vi "Random Seas.vi"() -> ()   [LabVIEW 2012]
uses:
  <vilib>/Daq/1easyio.llb/AO Update Channel (scaled value).vi
  Instance           1 19Saved   Random Seas .vi
  Instance           2 19Saved   Random Seas .vi
panel:
  out "File Name Out":path
  out "Wavestaff Signal":dbl[](graph)
  in  "Measure Waves":bool
  in  "Input Settings":bool
  in  "Geometric Settings":bool
  in  "Limit Settings":bool
  in  "Output Settings":bool
  out "Output Sig. Wave Height":dbl format="%.4f"
  out "Buffer Completed":dbl format="%.1f"
  out "Time Series Data":dbl[](array[numeric]) format="%.2f"
  out "Output Signal":dbl[](graph)
  in  "Set spectal parameters":bool
  in  "Run":bool
  in  "Power":bool
  out "Significant Wave Period":dbl format="%.4f"
  out "Significant Wave Height":dbl format="%.4f"
  in  "Select spectrum":u16(ring) items=["Bretschnieder", "JONSWAP", "NH Extreme", "NH Typical", "Pierson Moskowitz"]
  out "Spectra":cluster{"Numeric":dbl, "Numeric":dbl}[](graph)
  out "Time Series":cluster{"Numeric":dbl, "Numeric":sgl}[](graph)
  # "Random Sea Generator"
  # "m"
  # "s"
  # "Time (min:sec)"
  # "%"
  # "m"
  # "Time (min:sec)"
  # "Frequency (Hz)"
  # "Advanced"
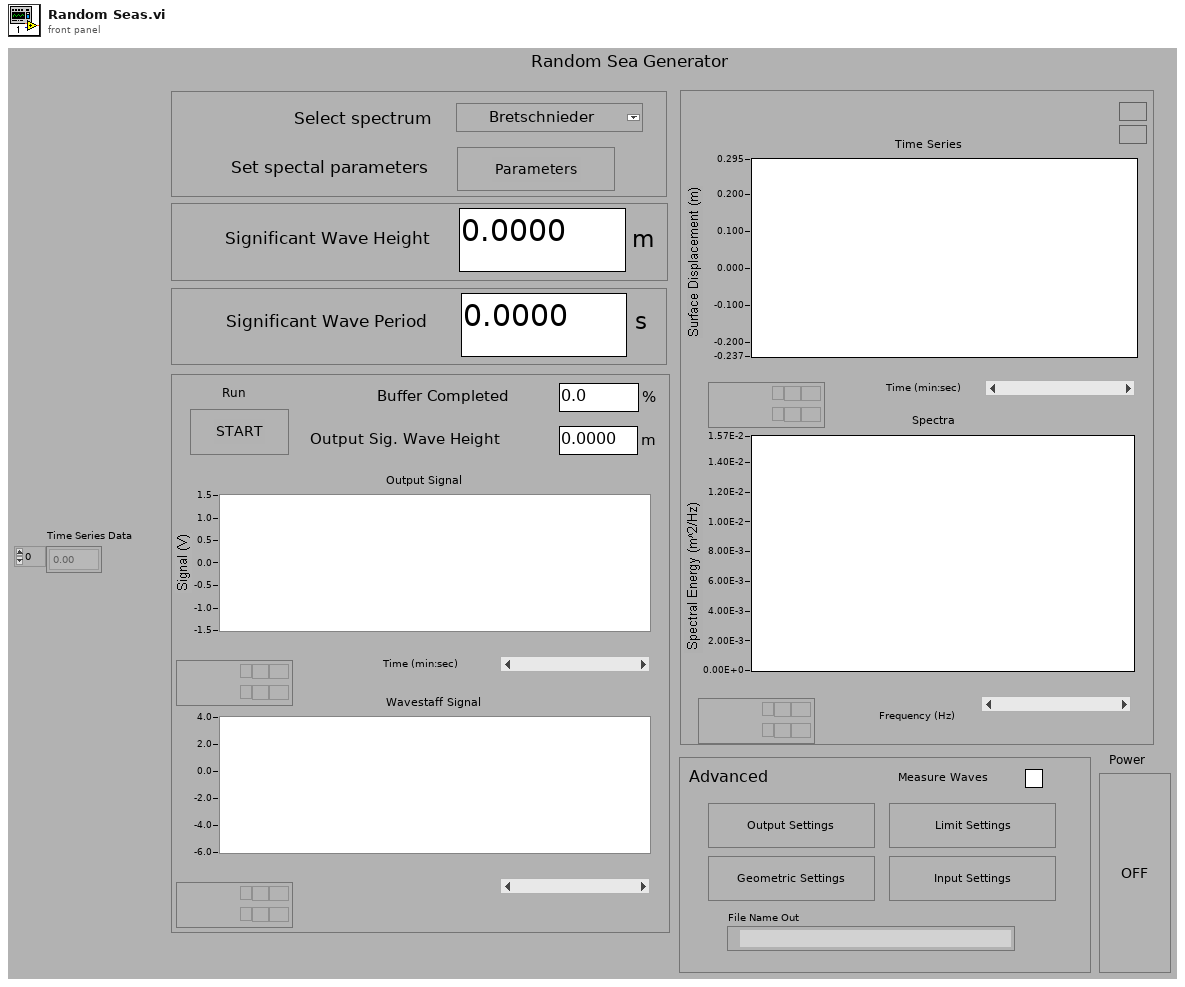
[diagram p1: front panel]
types:
  T1 = cluster{"Input Device":i32, "Input Channel":string, "Input Offset":dbl, "Input Calibration":dbl}
  T2 = cluster{"Device":i16, "Channel":string, "Sampling Rate":i32, "Ramp Time":dbl, "Buffer Length":u16, "Buffer Size":i32, "Sub Buffer Length":i16, "Sub Buffer Size":i16}
  T3 = cluster{"Stroke Calibration":dbl, "Water Depth":dbl, "Paddle Height":dbl}
  T4 = cluster{"Min Wave Period":dbl, "Max Wave Period":dbl, "Cutoff Frequency":dbl, "Max 1/2 Piston Stroke":dbl, "Max H/L":dbl, "Max H/d":dbl}
  T5 = cluster{"Bretschneider":cluster{"Sig Wave Height":dbl, "Sig Wave Period":dbl, "Scale Ratio":dbl}, "JONSWAP":cluster{"Sig Wave Height":dbl, "Sig Wave Period":dbl, "Gamma":dbl, "Sigma A":dbl, "Sigma B":dbl, "Scale Ratio":dbl}, "NH Extreme":cluster{"Sig Wave Height":dbl, "Sig Wave Period":dbl, "Gamma":dbl, "Sigma A":dbl, "Sigma B":dbl, "P":dbl, "Scale Ratio":dbl}, "NH Typical":cluster{"Sig Wave Height":dbl, "Sig Wave Period 1":dbl, "Sig Wave Period 2":dbl, "Gamma 1":dbl, "Gamma 2":dbl, "P":dbl, "Scale Ratio":dbl}, "PM":cluster{"Wind speed":dbl, "Scale Ratio":dbl}}
  T6 = cluster{"Element Data":dbl, "Element Data":dbl}[]
  T7 = cluster{"Sig Wave Height":dbl, "Sig Wave Period":dbl, "Scale Ratio":dbl}
  T8 = cluster{"Sig Wave Height":dbl, "Sig Wave Period":dbl, "Gamma":dbl, "Sigma A":dbl, "Sigma B":dbl, "Scale Ratio":dbl}
  T9 = cluster{"Sig Wave Height":dbl, "Sig Wave Period":dbl, "Gamma":dbl, "Sigma A":dbl, "Sigma B":dbl, "P":dbl, "Scale Ratio":dbl}
  T10 = cluster{"Sig Wave Height":dbl, "Sig Wave Period":dbl, "Sig Wave Period 2":dbl, "Gamma 1":dbl, "Gamma 2":dbl, "P":dbl, "Scale Ratio":dbl}
  T11 = cluster{"Device":i16, "Channel":string, "Sampling Rate":i32, "Stroke Calibration":dbl, "Buffer Length":u16, "Buffer Size":i32, "Sub Buffer Length":i16, "Sub Buffer Size":i16}
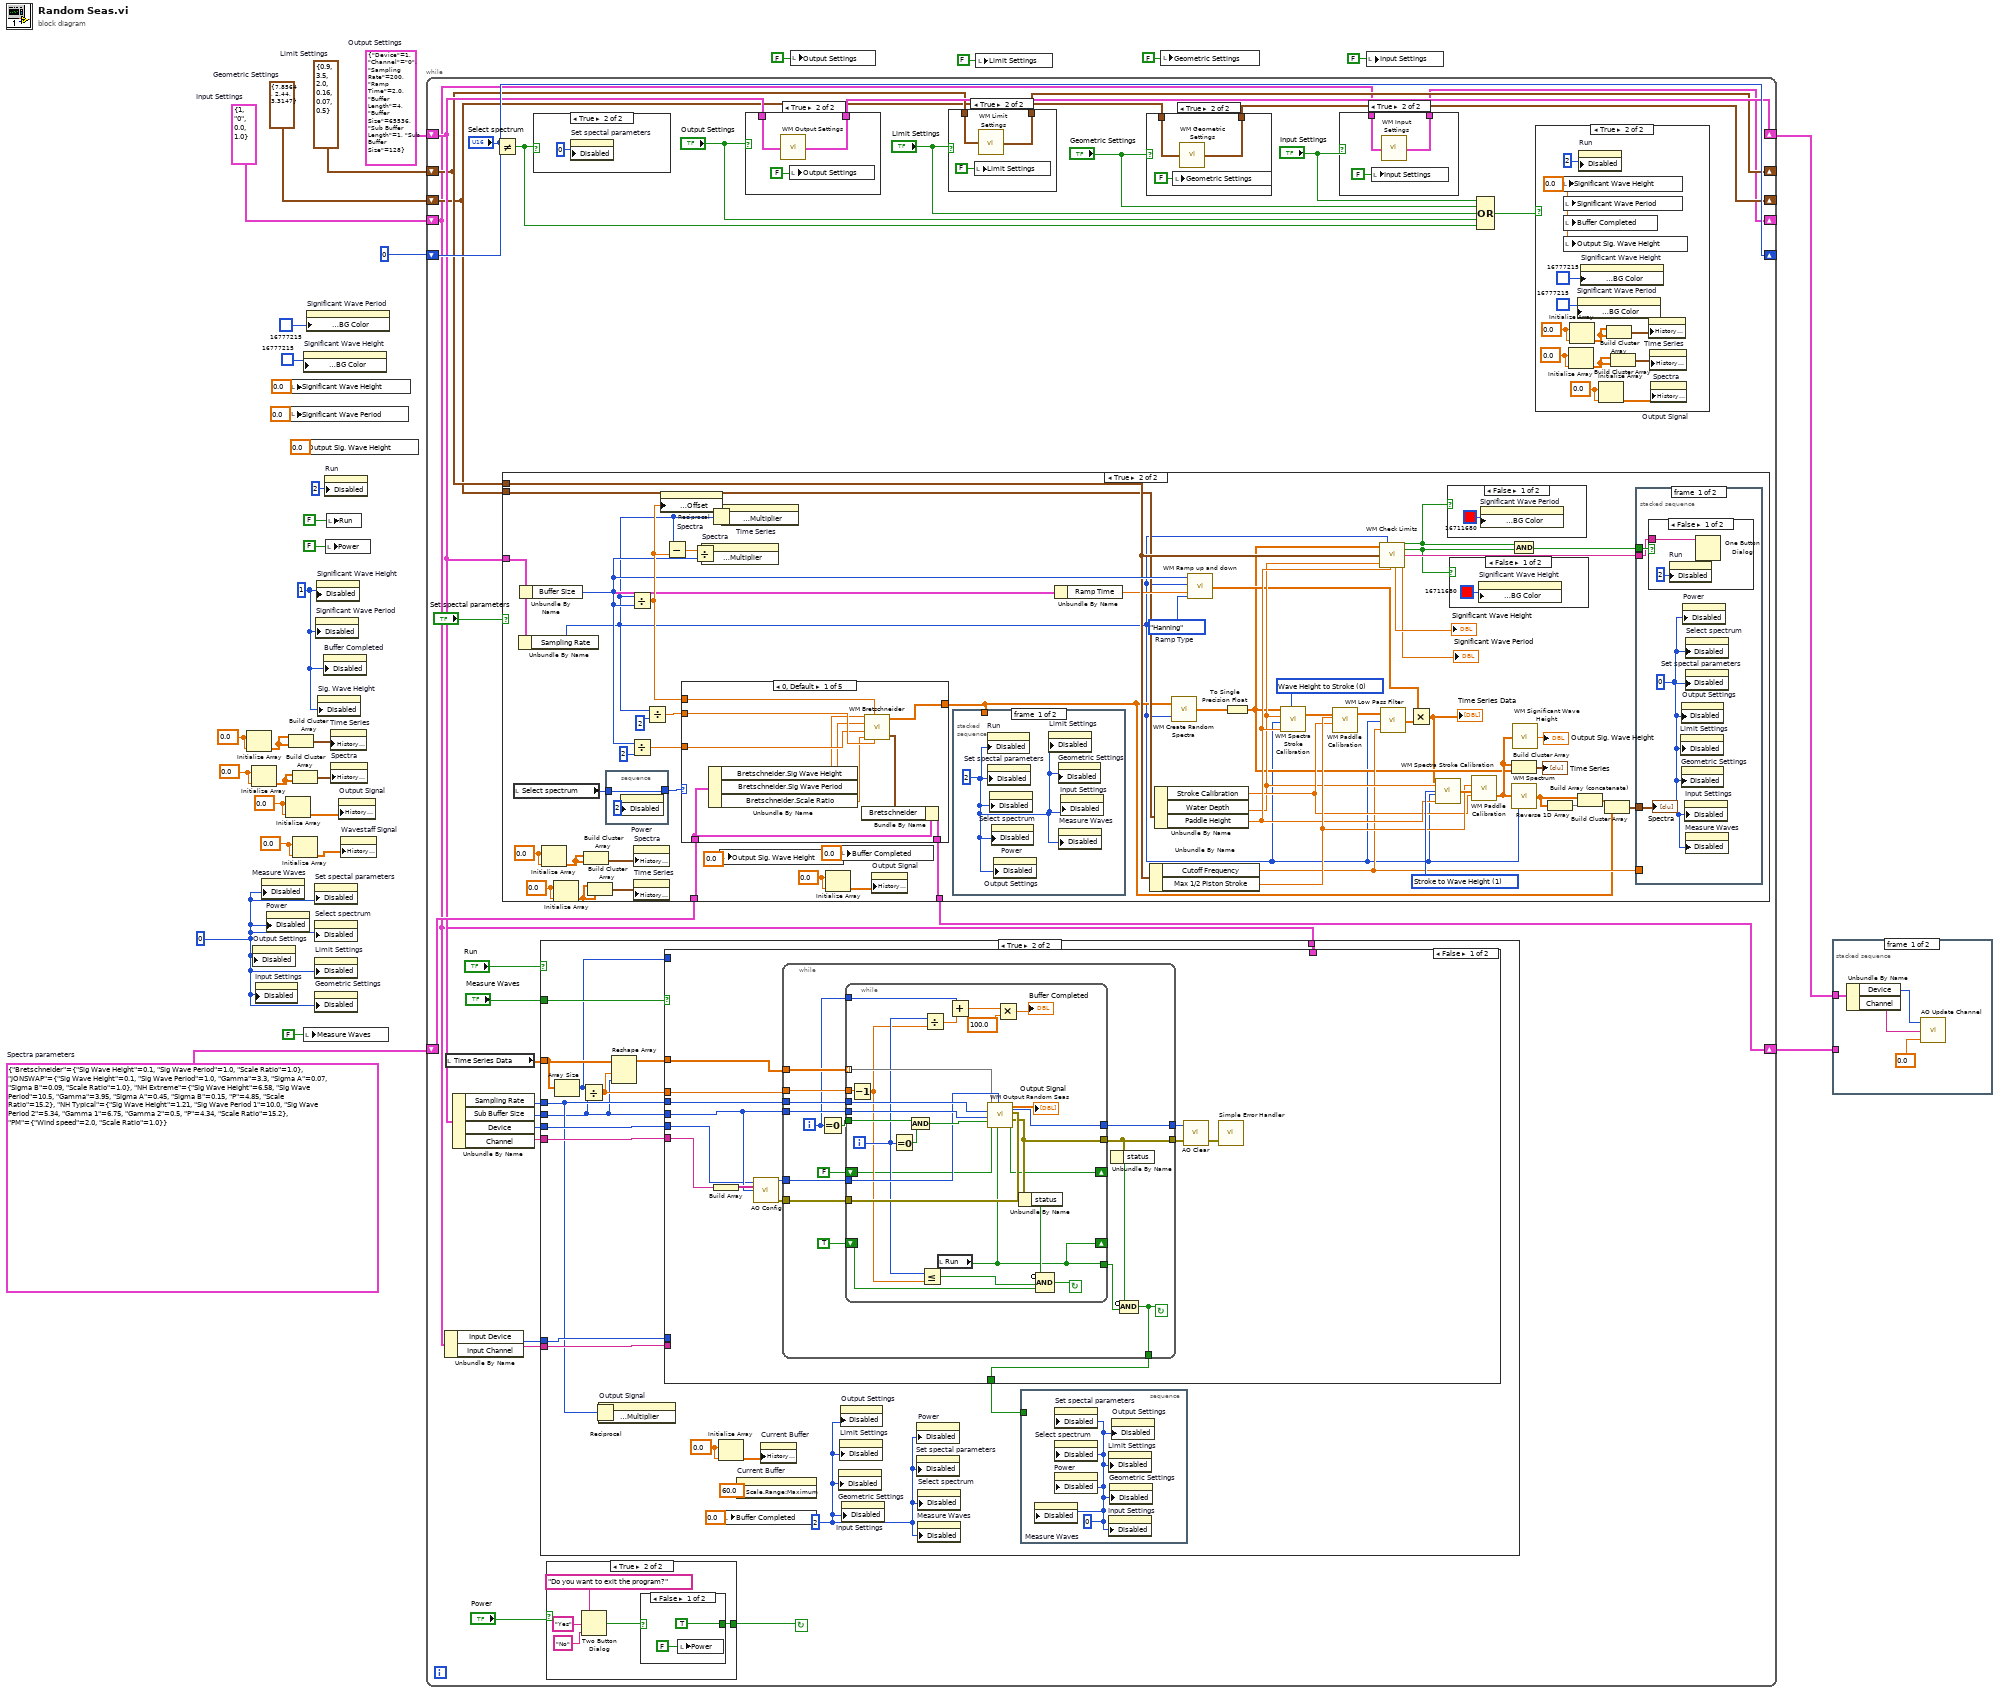
[diagram p0: block diagram]
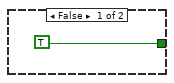
[diagram p7: hidden frame]
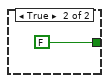
[diagram p8: hidden frame]
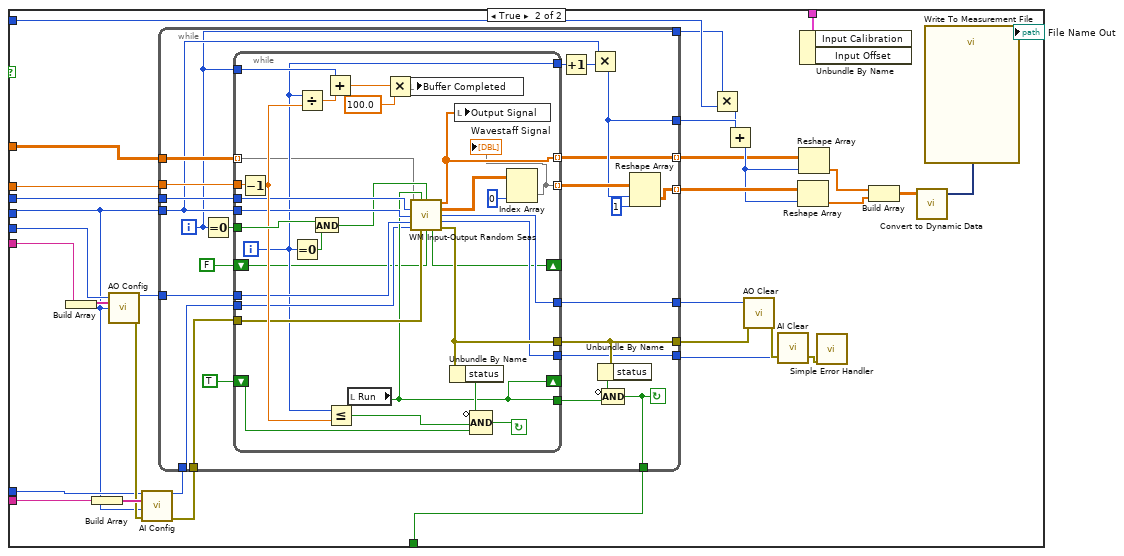
[diagram p11: hidden frame]
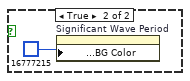
[diagram p13: hidden frame]
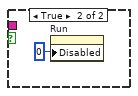
[diagram p15: hidden frame]
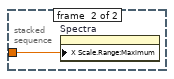
[diagram p16: hidden frame]
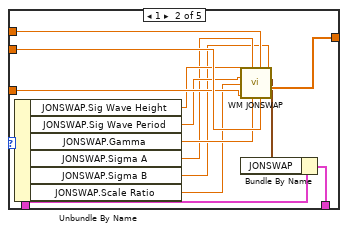
[diagram p17: hidden frame]
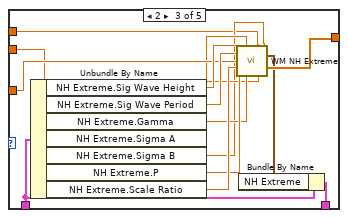
[diagram p18: hidden frame]
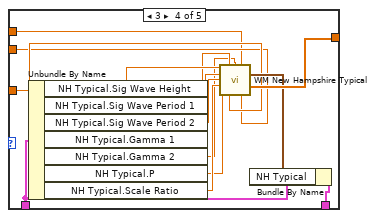
[diagram p19: hidden frame]
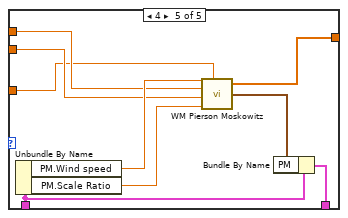
[diagram p20: hidden frame]
diagram:
  w2 = 0.0 ("Element Data")
  w5 = T1 {"Input Device"=1, "Input Channel"="0", "Input Offset"=0.0, "Input Calibration"=1.0}  # Input Settings
  w8 = T2 {"Device"=1, "Channel"="0", "Sampling Rate"=200, "Ramp Time"=2.0, "Buffer Length"=4, "Buffer Size"=65536, "Sub Buffer Length"=1, "Sub Buffer Size"=128}  # Output Settings
  w10 = T3 {"Stroke Calibration"=7.8564, "Water Depth"=2.44, "Paddle Height"=3.3147}  # Geometric Settings
  w11 = T4 {"Min Wave Period"=0.9, "Max Wave Period"=3.5, "Cutoff Frequency"=2.0, "Max 1/2 Piston Stroke"=0.16, "Max H/L"=0.07, "Max H/d"=0.5}  # Limit Settings
  w18 = 0.0 ("Element Data")
  w3 = u8 0 ("Write Attribute")
  w29 = 0.0 ("Element Data")
  w30 = 0.0 ("Element Data")
  w27 = T5 {"Bretschneider"={"Sig Wave Height"=0.1, "Sig Wave Period"=1.0, "Scale Ratio"=1.0}, "JONSWAP"={"Sig Wave Height"=0.1, "Sig Wave Period"=1.0, "Gamma"=3.3, "Sigma A"=0.07, "Sigma B"=0.09, "Scale Ratio"=1.0}, "NH Extreme"={"Sig Wave Height"=6.58, "Sig Wave Period"=10.5, "Gamma"=3.95, "Sigma A"=0.45, "Sigma B"=0.15, "P"=4.85, "Scale Ratio"=15.2}, "NH Typical"={"Sig Wave Height"=1.21, "Sig Wave Period 1"=10.0, "Sig Wave Period 2"=5.34, "Gamma 1"=6.75, "Gamma 2"=0.5, "P"=4.34, "Scale Ratio"=15.2}, "PM"={"Wind speed"=2.0, "Scale Ratio"=1.0}}  # Spectra parameters
  w9 = 1
  n1 = Initialize Array(w30, w30) -> (w20:dbl[])
  n2 = Initialize Array(w29, w29) -> (w28:dbl[])
  n3 = property on="Output Settings" class="Bool (strict)"("Disabled"=w3) -> ()  [unwired: 2 in, 2 out]
  n4 = property on="Input Settings" class="Bool (strict)"("Disabled"=w3) -> ()  [unwired: 2 in, 2 out]
  n5 = property on="Measure Waves" class="Bool (strict)"("Disabled"=w3) -> ()  [unwired: 2 in, 2 out]
  n6 = property on="Power" class="Bool (strict)"("Disabled"=w3) -> ()  [unwired: 2 in, 2 out]
  n7 = Initialize Array(w18, w18) -> (w17:dbl[])
  n8 = local write "Significant Wave Height"(0.0 ("Significant Wave Height")) -> ()
  n9 = local write "Significant Wave Period"(0.0 ("Significant Wave Period")) -> ()
  n10 = Build Cluster Array(w20, w20) -> (w19:T6)
  n11 = Initialize Array(w2, w2) -> (w1:dbl[])
  n12 = Build Cluster Array(w28, w28) -> (w21:T6)
  n13 = local write "Output Sig. Wave Height"(0.0 ("Sig. Wave Height")) -> ()
  n14 = property on="Significant Wave Height" class="DigNum (strict)"("Numeric Text.Text Colors:BG Color"=u32 16777215) -> ()  [unwired: 2 in, 2 out]
  n15 = local write "Measure Waves"(FALSE ("Measure Waves")) -> ()
  n16 = property on="Significant Wave Period" class="DigNum (strict)"("Numeric Text.Text Colors:BG Color"=u32 16777215) -> ()  [unwired: 2 in, 2 out]
  n17 = property on="Set spectal parameters" class="Bool"("Disabled"=w3) -> ()  [unwired: 2 in, 2 out]
  n18 = property on="Select spectrum" class="Ring (strict)"("Disabled"=w3) -> ()  [unwired: 2 in, 2 out]
  n19 = property on="Limit Settings" class="Bool (strict)"("Disabled"=w3) -> ()  [unwired: 2 in, 2 out]
  n20 = property on="Geometric Settings" class="Bool (strict)"("Disabled"=w3) -> ()  [unwired: 2 in, 2 out]
  n21 = property on="Significant Wave Period" class="DigNum (strict)"("Disabled"=w9) -> ()  [unwired: 2 in, 2 out]
  n22 = property on="Significant Wave Height" class="DigNum (strict)"("Disabled"=w9) -> ()  [unwired: 2 in, 2 out]
  n23 = property on="Sig. Wave Height" class="DigNum (strict)"("Disabled"=w9) -> ()  [unwired: 2 in, 2 out]
  n24 = property on="Buffer Completed" class="DigNum (strict)"("Disabled"=w9) -> ()  [unwired: 2 in, 2 out]
  n25 = property on="Run" class="Bool (strict)"("Disabled"=u8 2 ("Write Attribute")) -> ()  [unwired: 2 in, 2 out]
  n26 = local write "Power"(FALSE ("Power")) -> ()
  n27 = local write "Run"(FALSE ("Run")) -> ()
  n28 = property on="Time Series" class="WFChart (strict)"("History Data"=w19) -> ()  [unwired: 2 in, 2 out]
  n29 = property on="Spectra" class="WFChart (strict)"("History Data"=w21) -> ()  [unwired: 2 in, 2 out]
  n30 = property on="Output Signal" class="WFChart (strict)"("History Data"=w17) -> ()  [unwired: 2 in, 2 out]
  n31 = property on="Wavestaff Signal" class="WFChart (strict)"("History Data"=w1) -> ()  [unwired: 2 in, 2 out]
  n32 = while {
    shift-left: w5 -> [w34]
    shift-right: [w44] -> _
    shift-left: w10 -> [w45]
    shift-right: [w46] -> _
    shift-left: w11 -> [w47]
    shift-right: [w48] -> _
    shift-left: w8 -> [w53]
    shift-right: [w54] -> w14
    shift-left: 0 -> [w57]
    shift-right: ["Select spectrum"] -> _
    shift-left: w27 -> [w62]
    shift-right: [w61] -> w16
    stop <- w56 continue-if-true
    n33 = Unbundle By Name(w34) -> ("Input Device"=w36:i32, "Input Channel"=w35:string)
    n34 = local read "Time Series Data"() -> (w60:dbl[])
    n35 = Unbundle By Name(w53) -> ("Sampling Rate"=w52:i32, "Sub Buffer Size"=w51:i16, "Device"=w50:i16, "Channel"=w49:string)
    n36 = Not Equal?(x="Select spectrum", y=w57) -> (x != y?=w43:bool)
    n37 = case shown="True" "Set spectal parameters" {
      tunnel: [w264 w288] -> w61
      tunnel: w62 -> [w264 w312]
      tunnel: w53 -> [_ w275]
      tunnel: w47 -> [_ w279]
      tunnel: w45 -> [_ w277]
      frame False {
      }
      frame True {
        w286 = u16 0 items=["Wave Height to Stroke", "Stroke to Wave Height"] ("Conversion Type")
        w287 = u16 1 items=["Wave Height to Stroke", "Stroke to Wave Height"] ("Conversion Type")
        w311 = enum16{"Linear", "Hanning"}."Hanning"  # Ramp Type
        w297 = 0.0 ("Element Data")
        w309 = 0.0 ("Element Data")
        w319 = 0.0 ("Element Data")
        n38 = local read "Select spectrum"() -> (w299:u16)
        n39 = Unbundle By Name(w275) -> ("Sampling Rate"=w265:i32)
        n40 = Unbundle By Name(w275) -> ("Buffer Size"=w289:i32)
        n41 = Initialize Array(w309, w309) -> (w308:dbl[])
        n42 = Initialize Array(w319, w319) -> (w306:dbl[])
        n43 = Build Cluster Array(w308, w308) -> (w307:T6)
        n44 = Build Cluster Array(w306, w306) -> (w305:T6)
        n45 = stacked-sequence {
          tunnel: w299 -> [w326]
          tunnel: [w326] -> w298
          frame #0 {
            n46 = property on="Power" class="Bool (strict)"("Disabled"=u8 2 ("Write Attribute")) -> ()  [unwired: 2 in, 2 out]
          }
        }
        n47 = Divide(x=w265, y=w289) -> (x/y=w316:dbl)
        n48 = Divide(x=w289, y=2) -> (x/y=w318:dbl)
        n49 = property on="Spectra" class="WFChart (strict)"("History Data"=w307) -> ()  [unwired: 2 in, 2 out]
        n50 = property on="Time Series" class="WFChart (strict)"("History Data"=w305) -> ()  [unwired: 2 in, 2 out]
        n51 = Divide(x=w265, y=i8 2) -> (x/y=w317:dbl)
        n52 = property on="Spectra" class="WFChart (strict)"("X Scale.Offset and Multiplier:Offset"=w316) -> ()  [unwired: 2 in, 2 out]
        n53 = Subtract(x=w265, y=w316) -> (x-y=w320:dbl)
        n54 = case shown="0, Default" w298 {
          tunnel: [w345 w355 w362 w386 w392] -> w267
          tunnel: w318 -> [w342 w356 w370 w375 w387]
          tunnel: w317 -> [w343 w357 w366 w374 w388]
          tunnel: w316 -> [w344 w358 w363 w373 w389]
          tunnel: [w338 w346 w360 w385 w394] -> w288
          tunnel: w312 -> [w340 w348 w361 w383 w395]
          frame 0, Default {
            n55 = Unbundle By Name(w340) -> ("Bretschneider.Sig Wave Height"=w337:dbl, "Bretschneider.Sig Wave Period"=w336:dbl, "Bretschneider.Scale Ratio"=w341:dbl)
            n56 = call "WM Bretschneider.vi"("Significant Wave Height"=w337, "Start Freq"=w344, "Peak Wave Period"=w336, "Number of Frequencies"=w342, "End Freq"=w343, "Scale Ratio"=w341) -> ("Spectral Energy"=w345:dbl[], "Bretschneider parameters"=w339:T7)  [unwired: 1 out]
            n57 = Bundle By Name(cluster=w340, "Bretschneider"=w339) -> (w338:T5)
          }
          frame 1 {
            n58 = Unbundle By Name(w348) -> ("JONSWAP.Sig Wave Height"=w354:dbl, "JONSWAP.Sig Wave Period"=w353:dbl, "JONSWAP.Gamma"=w352:dbl, "JONSWAP.Sigma A"=w351:dbl, "JONSWAP.Sigma B"=w350:dbl, "JONSWAP.Scale Ratio"=w349:dbl)
            n59 = call "WM JONSWAP.vi"("Sigma B"=w350, "End Freq (Model Scale)"=w357, "Start Freq (Model Scale)"=w358, "Gamma"=w352, "Sigma A"=w351, "Number of Frequencies"=w356, "Scale Ratio"=w349, "Peak Wave Period"=w353, "Significant Wave Height"=w354) -> ("Spectral Energy"=w355:dbl[], "JONSWAP parameters"=w347:T8)  [unwired: 1 out]
            n60 = Bundle By Name(cluster=w348, "JONSWAP"=w347) -> (w346:T5)
          }
          frame 2 {
            n61 = Unbundle By Name(w361) -> ("NH Extreme.Sig Wave Height"=w372:dbl, "NH Extreme.Sig Wave Period"=w371:dbl, "NH Extreme.Gamma"=w367:dbl, "NH Extreme.Sigma A"=w365:dbl, "NH Extreme.Sigma B"=w364:dbl, "NH Extreme.P"=w368:dbl, "NH Extreme.Scale Ratio"=w369:dbl)
            n62 = call "WM NH Extreme.vi"("Significant Wave Height"=w372, "Sigma A"=w365, "Start Freq (Model Scale)"=w363, "Sigma B"=w364, "Peak Wave Period"=w371, "Number of Frequencies"=w370, "Scale Ratio"=w369, "P"=w368, "Gamma"=w367, "End Freq (Model Scale)"=w366) -> ("NH Extreme parameters"=w359:T9, "Spectral Energy"=w362:dbl[])  [unwired: 3 in, 1 out]
            n63 = Bundle By Name(cluster=w361, "NH Extreme"=w359) -> (w360:T5)
          }
          frame 3 {
            n64 = Unbundle By Name(w383) -> ("NH Typical.Sig Wave Height"=w382:dbl, "NH Typical.Sig Wave Period 1"=w381:dbl, "NH Typical.Sig Wave Period 2"=w380:dbl, "NH Typical.Gamma 1"=w377:dbl, "NH Typical.Gamma 2"=w376:dbl, "NH Typical.P"=w378:dbl, "NH Typical.Scale Ratio"=w379:dbl)
            n65 = call "WM New Hampshire Typical.vi"("Significant Wave Height"=w382, "Gamma 1"=w377, "Gamma 2"=w376, "Start Freq (Model Scale)"=w373, "Peak Wave Period 1"=w381, "Peak Wave Period 2"=w380, "Scale Ratio"=w379, "P"=w378, "Number of Frequencies"=w375, "End Freq (Model Scale)"=w374) -> ("NH Typical parameters"=w384:T10, "Spectral Energy"=w386:dbl[])  [unwired: 3 in, 1 out]
            n66 = Bundle By Name(cluster=w383, "NH Typical"=w384) -> (w385:T5)
          }
          frame 4 {
            n67 = Unbundle By Name(w395) -> ("PM.Wind speed"=w391:dbl, "PM.Scale Ratio"=w390:dbl)
            n68 = call "WM Pierson Moskowitz.vi"("Wind Speed"=w391, "Start Freq (Model Scale)"=w389, "End Freq (Model Scale)"=w388, "Scale Ratio"=w390, "Number of Frequencies"=w387) -> ("Spectral Energy"=w392:dbl[], "PM parameters"=w393:cluster{"Wind Speed":dbl, "Scale Ratio":dbl})  [unwired: 1 out]
            n69 = Bundle By Name(cluster=w395, "PM"=w393) -> (w394:T5)
          }
        }
        n70 = Divide(x=w320, y=w289) -> (x/y=w315:dbl)
        n71 = property on="Spectra" class="WFChart (strict)"("X Scale.Offset and Multiplier:Multiplier"=w315) -> ()  [unwired: 2 in, 2 out]
        n72 = Reciprocal(x=w265) -> (1/x=w294:dbl)
        n73 = local write "Output Sig. Wave Height"(0.0 ("Sig. Wave Height")) -> ()
        n74 = property on="Time Series" class="WFChart (strict)"("X Scale.Offset and Multiplier:Multiplier"=w294) -> ()  [unwired: 2 in, 2 out]
        n75 = Initialize Array(w297, w297) -> (w296:dbl[])
        n76 = local write "Buffer Completed"(0.0 ("Buffer Completed")) -> ()
        n77 = property on="Output Signal" class="WFChart (strict)"("History Data"=w296) -> ()  [unwired: 2 in, 2 out]
        n78 = stacked-sequence {
          tunnel: w267 -> [_ _]
          frame #0 {
            w327 = u8 2 ("Write Attribute")
            n79 = property on="Run" class="Bool (strict)"("Disabled"=w327) -> ()  [unwired: 2 in, 2 out]
            n80 = property on="Set spectal parameters" class="Bool"("Disabled"=w327) -> ()  [unwired: 2 in, 2 out]
            n81 = property on="Select spectrum" class="Ring (strict)"("Disabled"=w327) -> ()  [unwired: 2 in, 2 out]
            n82 = property on="Power" class="Bool (strict)"("Disabled"=w327) -> ()  [unwired: 2 in, 2 out]
            n83 = property on="Output Settings" class="Bool (strict)"("Disabled"=w327) -> ()  [unwired: 2 in, 2 out]
            n84 = property on="Limit Settings" class="Bool (strict)"("Disabled"=w327) -> ()  [unwired: 2 in, 2 out]
            n85 = property on="Geometric Settings" class="Bool (strict)"("Disabled"=w327) -> ()  [unwired: 2 in, 2 out]
            n86 = property on="Measure Waves" class="Bool (strict)"("Disabled"=w327) -> ()  [unwired: 2 in, 2 out]
            n87 = property on="Input Settings" class="Bool (strict)"("Disabled"=w327) -> ()  [unwired: 2 in, 2 out]
          }
          frame #1 {
          }
        }
        n88 = Unbundle By Name(w275) -> ("Ramp Time"=w278:dbl)
        n89 = Unbundle By Name(w279) -> ("Cutoff Frequency"=w271:dbl, "Max 1/2 Piston Stroke"=w280:dbl)
        n90 = Unbundle By Name(w277) -> ("Stroke Calibration"=w274:dbl, "Water Depth"=w273:dbl, "Paddle Height"=w276:dbl)
        n91 = call "WM Create Random Spectra.vi"("Sampling Freq"=w265, "Wave Spectra"=w267) -> ("Time Series"=w270:dbl[])
        n92 = call "WM Ramp up and down.vi"("Ramp Type"=w311, "Ramp Time"=w278, "Sampling Rate"=w265, "Buffer Size"=w289) -> ("Output"=w269:dbl[])
        n93 = To Single Precision Float(number=w270) -> (single precision float=w268:sgl[])
        n94 = call "WM Spectra Stroke Calibration.vi"("Input Time Series"=w268, "Water Depth"=w273, "Sampling Rate"=w265, "Paddle Height"=w276, "Conversion Type"=w286) -> ("Output Time Series"=w304:dbl[])
        n95 = call "WM Paddle Calibration.vi"("Stroke Calibration (V/m)"=w274, "Max 1/2 Piston Stroke (m)"=w280, "Input Stroke Distance (m)"=w304) -> ("Output Voltage"=w303:dbl[])  [unwired: 1 in, 1 out]
        n96 = call "WM Check Limits.vi"("Input Time Series"=w268, "Sampling Rate (Hz)"=w265, "Limit Settings"=w279, "Water Depth (m)"=w273, "Paddle Height (m)"=w276) -> ("Wave Period OK"=w282:bool, "Wave Height OK"=w283:bool, "Error Message"=w293:string, "Significant Wave Height (m)"=→"Significant Wave Height":dbl, "Significant Wave Period (s)"=→"Significant Wave Period":dbl)
        n97 = call "WM Low Pass Filter.vi"("Cutoff Freq"=w271, "Sampling Freq"=w265, "Input"=w303) -> ("Output"=w301:dbl[])
        n98 = Multiply(x=w269, y=w301) -> (x*y=w266:dbl[])
        "Time Series Data" <- w266
        n99 = call "WM Spectra Stroke Calibration.vi"("Input Time Series"=w266, "Water Depth"=w273, "Sampling Rate"=w265, "Paddle Height"=w276, "Conversion Type"=w287) -> ("Output Time Series"=w281:dbl[])
        n100 = case shown="False" w282 {
          frame False {
            n101 = property on="Significant Wave Period" class="DigNum (strict)"("Numeric Text.Text Colors:BG Color"=u32 16711680) -> ()  [unwired: 2 in, 2 out]
          }
          frame True {
            n102 = property on="Significant Wave Period" class="DigNum (strict)"("Numeric Text.Text Colors:BG Color"=u32 16777215) -> ()  [unwired: 2 in, 2 out]
          }
        }
        n103 = case shown="False" w283 {
          frame False {
            n104 = property on="Significant Wave Height" class="DigNum (strict)"("Numeric Text.Text Colors:BG Color"=u32 16711680) -> ()  [unwired: 2 in, 2 out]
          }
          frame True {
            n105 = property on="Significant Wave Height" class="DigNum (strict)"("Numeric Text.Text Colors:BG Color"=u32 16777215) -> ()  [unwired: 2 in, 2 out]
          }
        }
        n106 = call "WM Paddle Calibration.vi"("Input Voltage"=w281, "Stroke Calibration (V/m)"=w274, "Max 1/2 Piston Stroke (m)"=w280) -> ("Output Stroke Distance"=w292:dbl[])  [unwired: 1 in, 1 out]
        n107 = And(x=w282, y=w283) -> (x .and. y?=w300:bool)
        n108 = Build Cluster Array(w292, w268) -> (→"Time Series":cluster{"Numeric":dbl, "Numeric":sgl}[])
        n109 = call "WM Spectrum.vi"("Sampling Rate"=w265, "Time Series"=w292) -> ("Spectra"=w314:dbl[])
        n110 = call "WM Significant Wave Height.vi"("Input"=w292) -> ("Significant Wave Height"=→"Output Sig. Wave Height":dbl)
        n111 = Reverse 1D Array(array=w314) -> (reversed array=w313:dbl[])
        n112 = Build Array (concatenate)(w314, w313) -> (w310:dbl[])
        n113 = Build Cluster Array(w310, w267) -> (w272:cluster{"Numeric":dbl, dbl}[])
        n114 = stacked-sequence {
          tunnel: w272 -> [w331 _]
          tunnel: w300 -> [w330 _]
          tunnel: w293 -> [w329 _]
          tunnel: w271 -> [_ w335]
          frame #0 {
            w328 = u8 0 ("Write Attribute")
            n115 = case shown="False" w330 {
              tunnel: w329 -> [w332 _]
              frame False {
                n116 = property on="Run" class="Bool (strict)"("Disabled"=u8 2 ("Write Attribute")) -> ()  [unwired: 2 in, 2 out]
                n117 = One Button Dialog(message=w332) -> ()  [unwired: 1 in, 1 out]
              }
              frame True {
                n118 = property on="Run" class="Bool (strict)"("Disabled"=u8 0 ("Write Attribute")) -> ()  [unwired: 2 in, 2 out]
              }
            }
            n119 = property on="Limit Settings" class="Bool (strict)"("Disabled"=w328) -> ()  [unwired: 2 in, 2 out]
            n120 = property on="Output Settings" class="Bool (strict)"("Disabled"=w328) -> ()  [unwired: 2 in, 2 out]
            n121 = property on="Geometric Settings" class="Bool (strict)"("Disabled"=w328) -> ()  [unwired: 2 in, 2 out]
            n122 = property on="Power" class="Bool (strict)"("Disabled"=w328) -> ()  [unwired: 2 in, 2 out]
            n123 = property on="Input Settings" class="Bool (strict)"("Disabled"=w328) -> ()  [unwired: 2 in, 2 out]
            n124 = property on="Select spectrum" class="Ring (strict)"("Disabled"=w328) -> ()  [unwired: 2 in, 2 out]
            n125 = property on="Set spectal parameters" class="Bool"("Disabled"=w328) -> ()  [unwired: 2 in, 2 out]
            n126 = property on="Measure Waves" class="Bool (strict)"("Disabled"=w328) -> ()  [unwired: 2 in, 2 out]
            "Spectra" <- w331
          }
          frame #1 {
            n127 = property on="Spectra" class="WFChart (strict)"("X Scale.Range:Maximum"=w335) -> ()  [unwired: 2 in, 2 out]
          }
        }
      }
    }
    n128 = case shown="True" w43 {
      frame False {
      }
      frame True {
        n129 = property on="Set spectal parameters" class="Bool"("Disabled"=u8 0 ("Write Attribute")) -> ()  [unwired: 2 in, 2 out]
      }
    }
    n130 = case shown="True" "Run" {
      tunnel: w60 -> [_ w108]
      tunnel: w52 -> [_ w109]
      tunnel: w51 -> [_ w105]
      tunnel: w50 -> [_ w116]
      tunnel: w49 -> [_ w115]
      tunnel: "Measure Waves" -> [_ w114]
      tunnel: w36 -> [_ w113]
      tunnel: w35 -> [_ w112]
      tunnel: w34 -> [_ w104]
      frame False {
      }
      frame True {
        w103 = u8 2 ("Write Attribute")
        w120 = 0.0 ("Element Data")
        n131 = Array Size(array=w108) -> (size(s)=w102:i32)
        n132 = Divide(x=w102, y=w105) -> (x/y=w106:dbl)
        n133 = Reciprocal(x=w109) -> (1/x=w110:dbl)
        n134 = property on="Output Signal" class="WFChart (strict)"("X Scale.Offset and Multiplier:Multiplier"=w110) -> ()  [unwired: 2 in, 2 out]
        n135 = Reshape Array(w108, w106, w105) -> (w107:dbl[][])
        n136 = case shown="False" w114 {
          tunnel: w107 -> [w123 w191]
          tunnel: w109 -> [w127 w194]
          tunnel: w105 -> [w126 w187]
          tunnel: w116 -> [w125 w195]
          tunnel: w115 -> [w124 w196]
          tunnel: w113 -> [_ w197]
          tunnel: w112 -> [_ w200]
          tunnel: [w121 w189] -> w111
          tunnel: w106 -> [w122 w190]
          tunnel: w104 -> [_ w188]
          tunnel: w102 -> [_ w183]
          frame False {
            n137 = Build Array(w124) -> (w133:string[])
            n138 = call <vilib>:"AO Config.vi"("device (1)"=w125, "channels (0)"=w133, "buffer size (1000 updates)"=w126) -> ("taskID"=w132:u32, "error out"=w131:errorcluster)  [unwired: 10 in, 1 out]
            n139 = while {
              tunnel: [w140] -> w128
              tunnel: [w139] -> w129
              tunnel: w131 -> [w141]
              tunnel: w132 -> [w142]
              tunnel: w127 -> [w143]
              tunnel: [w144] -> w121
              tunnel: w122 -> [w146]
              tunnel: w126 -> [w148]
              tunnel: w123 -> [w147]
              i -> [w136]
              stop <- w144 continue-if-true
              n140 = Equal To 0?(x=w136) -> (x = 0?=w138:bool)
              n141 = while {
                shift-left: TRUE ("Run") -> [w149]
                shift-right: [w150] -> _
                shift-left: FALSE ("End Out") -> [w151]
                shift-right: [w152] -> _
                tunnel: w136 -> [w159]
                tunnel: [w162] -> w140
                tunnel: [w165] -> w139
                tunnel: w141 -> [w166]
                tunnel: w142 -> [w167]
                tunnel: w143 -> [w170]
                tunnel: [w150] -> w145
                tunnel: w146 -> [w172]
                tunnel: w147 -> [w160] mode=indexing
                tunnel: w138 -> [w173]
                tunnel: w148 -> [w171]
                i -> [w158]
                stop <- w169 continue-if-true
                n142 = Decrement(x=w172) -> (x-1=w156:dbl)
                n143 = Equal To 0?(x=w158) -> (x = 0?=w174:bool)
                n144 = And(x=w173, y=w174) -> (x .and. y?=w168:bool)
                n145 = Less Or Equal?(x=w158, y=w156) -> (x <= y?=w161:bool)
                n146 = Divide(x=w158, y=w156) -> (x/y=w157:dbl)
                n147 = local read "Run"() -> (w150:bool)
                n148 = Add(x=w159, y=w157) -> (x+y=w155:dbl)
                n149 = call "WM Output Random Seas.vi"("error in (no error)"=w166, "Start up"=w168, "Run"=w150, "Task ID In"=w167, "End"=w151, "Sub Buffer Size"=w171, "Sampling Rate"=w170, "Input Time Series"=w160) -> ("End Out"=w152:bool, "error out"=w165:errorcluster, "Buffer"=→"Output Signal":dbl[], "Task ID Out"=w162:u32)
                n150 = Multiply(x=w155, y=100.0) -> (x*y=→"Buffer Completed":dbl)
                n151 = Unbundle By Name(w165) -> ("status"=w164:bool)
                n152 = Compound Arithmetic op=AND(invert w164, w161, w149) -> (w169:bool)
              }
              n153 = Unbundle By Name(w139) -> ("status"=w137:bool)
              n154 = Compound Arithmetic op=AND(invert w137, w145) -> (w144:bool)
            }
            n155 = call <vilib>:"AO Clear.vi"("error in (no error)"=w129, "taskID in"=w128) -> ("error out"=w130:errorcluster)  [unwired: 4 in, 1 out]
            n156 = call <vilib>:"Simple Error Handler.vi"("error in (no error)"=w130) -> ()  [unwired: 4 in, 5 out]
          }
          frame True {
            n157 = Build Array(w196) -> (w207:string[])
            n158 = Build Array(w200) -> (w199:string[])
            n159 = call <vilib>:"AO Config.vi"("device (1)"=w195, "channels (0)"=w207, "buffer size (1000 updates)"=w187) -> ("taskID"=w206:u32, "error out"=w198:errorcluster)  [unwired: 10 in, 1 out]
            n160 = call <vilib>:"AI Config.vi"("device (1)"=w197, "channels (0)"=w199, "buffer size (1000 scans)"=w187, "error in (no error)"=w198) -> ("taskID"=w193:u32, "error out"=w192:errorcluster)  [unwired: 9 in, 1 out]
            n161 = while {
              tunnel: [w210] -> w186
              tunnel: [w213] -> w182
              tunnel: [w211] -> w185 mode=indexing
              tunnel: [w218] -> w201
              tunnel: w193 -> [w219]
              tunnel: w192 -> [w220]
              tunnel: [w224] -> w204
              tunnel: [w223] -> w205
              tunnel: w206 -> [w225]
              tunnel: w194 -> [w226]
              tunnel: [w227] -> w189
              tunnel: w190 -> [w229]
              tunnel: w187 -> [w215]
              tunnel: w191 -> [w231]
              tunnel: [w208] -> w179 mode=indexing
              i -> [w213]
              stop <- w227 continue-if-true
              n162 = Equal To 0?(x=w213) -> (x = 0?=w222:bool)
              n163 = while {
                shift-left: FALSE ("End Out") -> [w235]
                shift-right: [w236] -> _
                tunnel: [w238] -> w217
                tunnel: [w232] -> w212 mode=indexing
                tunnel: [w241] -> w218
                tunnel: w219 -> [w245]
                tunnel: w213 -> [w255]
                tunnel: [w243] -> w224
                tunnel: [w242] -> w223
                tunnel: w220 -> [w247]
                tunnel: w225 -> [w250]
                tunnel: w226 -> [w249]
                tunnel: [w246] -> w228
                tunnel: w229 -> [w259]
                shift-left: TRUE ("StartStop") -> [w260]
                shift-right: [w246] -> _
                tunnel: w231 -> [w234] mode=indexing
                tunnel: w222 -> [w261]
                tunnel: w215 -> [w248]
                tunnel: [w233] -> w208 mode=indexing
                i -> [w238]
                stop <- w258 continue-if-true
                n164 = Decrement(x=w259) -> (x-1=w253:dbl)
                n165 = Equal To 0?(x=w238) -> (x = 0?=w262:bool)
                n166 = Divide(x=w238, y=w253) -> (x/y=w254:dbl)
                n167 = And(x=w261, y=w262) -> (x .and. y?=w244:bool)
                n168 = Add(x=w255, y=w254) -> (x+y=w252:dbl)
                n169 = Less Or Equal?(x=w238, y=w253) -> (x <= y?=w256:bool)
                n170 = local read "Run"() -> (w246:bool)
                n171 = Multiply(x=w252, y=100.0) -> (x*y=w240:dbl)
                n172 = local write "Buffer Completed"(w240) -> ()
                n173 = call "WM Input-Output Random Seas.vi"("Output Time Series"=w234, "Run"=w246, "Start up/Continue"=w244, "Sampling Rate"=w249, "Sub Buffer Size"=w248, "Output Task ID In"=w250, "Input Task ID In"=w245, "error in (no error)"=w247, "End"=w235) -> ("Buffer"=w233:dbl[], "Experimental Data"=w237:dbl[][], "Output Task ID Out"=w243:u32, "Input Task ID Out"=w241:u32, "End Out"=w236:bool, "error out"=w242:errorcluster)  [unwired: 1 in]
                n174 = Unbundle By Name(w242) -> ("status"=w257:bool)
                n175 = local write "Output Signal"(w233) -> ()
                n176 = Compound Arithmetic op=AND(invert w257, w256, w260) -> (w258:bool)
                n177 = Index Array(array=w237, index (col)=0 ("Index")) -> (element=w232:dbl[])  [unwired: 1 in]
                "Wavestaff Signal" <- w232
              }
              n178 = Increment(x=w217) -> (x+1=w216:i32)
              n179 = Multiply(x=w215, y=w216) -> (x*y=w210:i32)
              n180 = Unbundle By Name(w223) -> ("status"=w221:bool)
              n181 = Compound Arithmetic op=AND(invert w221, w228) -> (w227:bool)
              n182 = Reshape Array(w212, w210, 1 ("Dimension Size")) -> (w211:dbl[][])
            }
            n183 = Multiply(x=w182, y=w183) -> (x*y=w184:i32)
            n184 = Add(x=w184, y=w186) -> (x+y=w180:i32)
            n185 = call <vilib>:"AO Clear.vi"("error in (no error)"=w205, "taskID in"=w204) -> ("error out"=w202:errorcluster)  [unwired: 4 in, 1 out]
            n186 = call <vilib>:"AI Clear.vi"("error in (no error)"=w202, "taskID in"=w201) -> ("error out"=w203:errorcluster)  [unwired: 4 in, 1 out]
            n187 = Reshape Array(w185, w180) -> (w181:dbl[])
            n188 = Reshape Array(w179, w180) -> (w178:dbl[])
            n189 = Unbundle By Name(w188) -> ()  [unwired: 2 out]
            n190 = call <vilib>:"Simple Error Handler.vi"("error in (no error)"=w203) -> ()  [unwired: 4 in, 5 out]
            n191 = Build Array(w178, w181) -> (w177:dbl[][])
            n192 = call "Convert to Dynamic Data"("2D Array"=w177) -> ("Dynamic Data Type"=w176:dynamicdata)  [unwired: 3 in]
            n193 = call "Write To Measurement File"("Signals"=w176) -> ("File Name Out"=→"File Name Out":path)  [unwired: 16 in, 2 out]
          }
        }
        n194 = Initialize Array(w120, w120) -> (w119:dbl[])
        n195 = local write "Buffer Completed"(0.0 ("Buffer Completed")) -> ()
        n196 = property on="Current Buffer" class="WFChart (strict)"("X Scale.Range:Maximum"=60.0 ("Write Attribute")) -> ()  [unwired: 2 in, 2 out]
        n197 = property on="Current Buffer" class="WFChart (strict)"("History Data"=w119) -> ()  [unwired: 2 in, 2 out]
        n198 = property on="Geometric Settings" class="Bool (strict)"("Disabled"=w103) -> ()  [unwired: 2 in, 2 out]
        n199 = property on="Limit Settings" class="Bool (strict)"("Disabled"=w103) -> ()  [unwired: 2 in, 2 out]
        n200 = property on="Output Settings" class="Bool (strict)"("Disabled"=w103) -> ()  [unwired: 2 in, 2 out]
        n201 = property on="Input Settings" class="Bool (strict)"("Disabled"=w103) -> ()  [unwired: 2 in, 2 out]
        n202 = property on="Power" class="Bool (strict)"("Disabled"=w103) -> ()  [unwired: 2 in, 2 out]
        n203 = property on="Set spectal parameters" class="Bool"("Disabled"=w103) -> ()  [unwired: 2 in, 2 out]
        n204 = property on="Select spectrum" class="Ring (strict)"("Disabled"=w103) -> ()  [unwired: 2 in, 2 out]
        n205 = property on="Measure Waves" class="Bool (strict)"("Disabled"=w103) -> ()  [unwired: 2 in, 2 out]
        n206 = stacked-sequence {
          tunnel: w111 -> [_]
          frame #0 {
            w263 = 0
            n207 = property on="Measure Waves" class="Bool (strict)"("Disabled"=w263) -> ()  [unwired: 2 in, 2 out]
            n208 = property on="Set spectal parameters" class="Bool"("Disabled"=w263) -> ()  [unwired: 2 in, 2 out]
            n209 = property on="Select spectrum" class="Ring (strict)"("Disabled"=w263) -> ()  [unwired: 2 in, 2 out]
            n210 = property on="Power" class="Bool (strict)"("Disabled"=w263) -> ()  [unwired: 2 in, 2 out]
            n211 = property on="Limit Settings" class="Bool (strict)"("Disabled"=w263) -> ()  [unwired: 2 in, 2 out]
            n212 = property on="Input Settings" class="Bool (strict)"("Disabled"=w263) -> ()  [unwired: 2 in, 2 out]
            n213 = property on="Geometric Settings" class="Bool (strict)"("Disabled"=w263) -> ()  [unwired: 2 in, 2 out]
            n214 = property on="Output Settings" class="Bool (strict)"("Disabled"=w263) -> ()  [unwired: 2 in, 2 out]
          }
        }
      }
    }
    n215 = case shown="True" "Power" {
      tunnel: [TRUE w93] -> w56
      frame False {
      }
      frame True {
        n216 = Two Button Dialog(message="Do you want to exit the program?", 1:"No" ("F button name (\"Cancel\")"), 2:"Yes" ("T button name (\"OK\")")) -> (T button?=w94:bool)
        n217 = case shown="False" w94 {
          tunnel: [TRUE FALSE] -> w93
          frame False {
            n218 = local write "Power"(FALSE ("Power")) -> ()
          }
          frame True {
          }
        }
      }
    }
    n219 = case shown="True" "Output Settings" {
      tunnel: w53 -> [w88 w89]
      tunnel: [w88 w91] -> w54
      frame False {
      }
      frame True {
        n220 = call "WM Output Settings.vi"("Output Settings"=w89) -> ("Output Settings Results"=w91:T11)
        n221 = local write "Output Settings"(FALSE ("Output Settings")) -> ()
      }
    }
    n222 = case shown="True" "Limit Settings" {
      tunnel: w47 -> [w84 w86]
      tunnel: [w84 w85] -> w48
      frame False {
      }
      frame True {
        n223 = local write "Limit Settings"(FALSE ("Limit Settings")) -> ()
        n224 = call "WM Limit Settings.vi"("Limit Settings"=w86) -> ("Limit Settings Output"=w85:T4)
      }
    }
    n225 = case shown="True" "Geometric Settings" {
      tunnel: w45 -> [w80 w83]
      tunnel: [w80 w82] -> w46
      frame False {
      }
      frame True {
        n226 = local write "Geometric Settings"(FALSE ("Geometric Settings")) -> ()
        n227 = call "WM Geometric Settings.vi"("Geometric Settings"=w83) -> ("Geometric Settings Output"=w82:T3)
      }
    }
    n228 = case shown="True" "Input Settings" {
      tunnel: w34 -> [w76 w77]
      tunnel: [w76 w78] -> w44
      frame False {
      }
      frame True {
        n229 = local write "Input Settings"(FALSE ("Input Settings")) -> ()
        n230 = call "WM Input Settings.vi"("Input Settings"=w77) -> ("Input Settings Out"=w78:T1)
      }
    }
    n231 = Compound Arithmetic op=OR("Input Settings", "Geometric Settings", "Limit Settings", "Output Settings", w43) -> (w38:bool)
    n232 = case shown="True" w38 {
      frame False {
      }
      frame True {
        w65 = 0.0 ("Element Data")
        w70 = 0.0 ("Element Data")
        w71 = 0.0 ("Element Data")
        w74 = 0.0 ("Significant Wave Height")
        n233 = local write "Significant Wave Height"(w74) -> ()
        n234 = local write "Significant Wave Period"(w74) -> ()
        n235 = local write "Buffer Completed"(w74) -> ()
        n236 = local write "Output Sig. Wave Height"(w74) -> ()
        n237 = Initialize Array(w70, w70) -> (w69:dbl[])
        n238 = Initialize Array(w71, w71) -> (w67:dbl[])
        n239 = property on="Significant Wave Period" class="DigNum (strict)"("Numeric Text.Text Colors:BG Color"=u32 16777215) -> ()  [unwired: 2 in, 2 out]
        n240 = property on="Run" class="Bool (strict)"("Disabled"=u8 2 ("Write Attribute")) -> ()  [unwired: 2 in, 2 out]
        n241 = property on="Significant Wave Height" class="DigNum (strict)"("Numeric Text.Text Colors:BG Color"=u32 16777215) -> ()  [unwired: 2 in, 2 out]
        n242 = Initialize Array(w65, w65) -> (w64:dbl[])
        n243 = Build Cluster Array(w67, w67) -> (w66:T6)
        n244 = Build Cluster Array(w69, w69) -> (w68:T6)
        n245 = property on="Time Series" class="WFChart (strict)"("History Data"=w66) -> ()  [unwired: 2 in, 2 out]
        n246 = property on="Spectra" class="WFChart (strict)"("History Data"=w68) -> ()  [unwired: 2 in, 2 out]
        n247 = property on="Output Signal" class="WFChart (strict)"("History Data"=w64) -> ()  [unwired: 2 in, 2 out]
      }
    }
  }
  n248 = local write "Output Settings"(FALSE ("Output Settings")) -> ()
  n249 = local write "Limit Settings"(FALSE ("Limit Settings")) -> ()
  n250 = local write "Geometric Settings"(FALSE ("Geometric Settings")) -> ()
  n251 = local write "Input Settings"(FALSE ("Input Settings")) -> ()
  n252 = stacked-sequence {
    tunnel: w16 -> [_ _]
    tunnel: w14 -> [w400 _]
    frame #0 {
      n253 = Unbundle By Name(w400) -> ("Device"=w399:i16, "Channel"=w398:string)
      n254 = call-poly <vilib>:"AO Update Channel.vi"("value"=sgl 0.0, "channel (0)"=w398, "device"=w399) -> ()
    }
    frame #1 {
      n255 = Quit LabVIEW() -> ()  [unwired: 1 in]
    }
  }
